vi "EQ make summary.vi"(4 "quants pixels bons per Chip":u8[](array[numeric])) -> (1 "summary EQ":string)   [LabVIEW 2015, in "VIPM2.lvlib"]
doc: "A partir de la llista de pixles bons per Chip, calcula el total de pixels bons i dolents amb els percentatges corresponents."
uses:
  VIPM2.lvlib
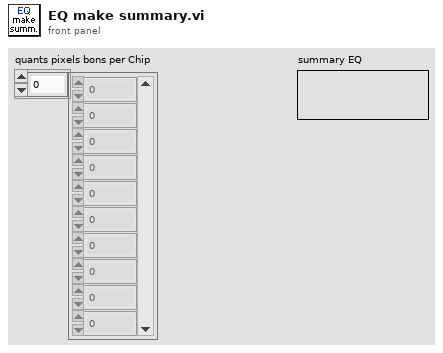
[diagram p1: front panel]
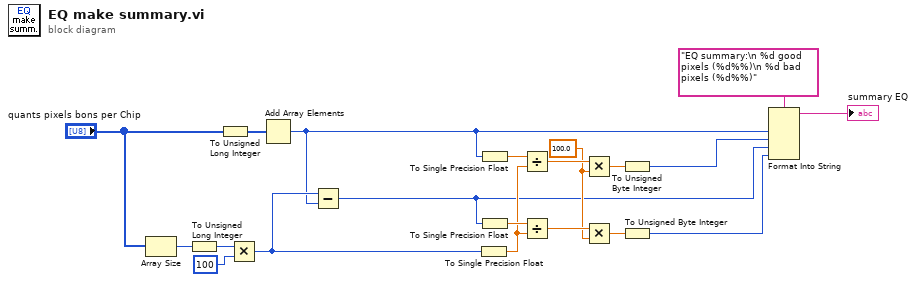
[diagram p0: block diagram]
diagram:
  w8 = sgl 100.0 ("y")
  n1 = Array Size(array="quants pixels bons per Chip") -> (size(s)=w16:i32)
  n2 = To Unsigned Long Integer(number=w16) -> (unsigned 32bit integer=w17:u32)
  n3 = To Unsigned Long Integer(number="quants pixels bons per Chip") -> (unsigned 32bit integer=w20:u32[])
  n4 = Multiply(x=w17, y=u32 100) -> (x*y=w15:u32)
  n5 = Add Array Elements(numeric array=w20) -> (sum=w6:u32)
  n6 = Subtract(x=w15, y=w6) -> (x-y=w4:u32)
  n7 = To Single Precision Float(number=w15) -> (single precision float=w7:sgl)
  n8 = To Single Precision Float(number=w6) -> (single precision float=w14:sgl)
  n9 = To Single Precision Float(number=w4) -> (single precision float=w9:sgl)
  n10 = Divide(x=w14, y=w7) -> (x/y=w13:sgl)
  n11 = Divide(x=w9, y=w7) -> (x/y=w10:sgl)
  n12 = Multiply(x=w13, y=w8) -> (x*y=w12:sgl)
  n13 = Multiply(x=w10, y=w8) -> (x*y=w11:sgl)
  n14 = To Unsigned Byte Integer(number=w12) -> (unsigned 8bit integer=w5:u8)
  n15 = To Unsigned Byte Integer(number=w11) -> (unsigned 8bit integer=w3:u8)
  n16 = Format Into String "Format Into String"(format string="EQ summary:\n %d good pixels (%d%%)\n %d bad pixels (%d%%)", w6, w5, w4, w3) -> (resulting string=→"summary EQ":string)  [unwired: 2 in, 1 out]
